vi "Post Webmessage.vi"(8 "error in (no error)":errorcluster, 9 "Send as JSON":bool, 10 "Message":string, 11 "WebView2 Control in":refnum<class "WebView2 Control.lvclass">) -> (0 "error out":errorcluster, 3 "WebView2 Control out":refnum<class "WebView2 Control.lvclass">)   [LabVIEW 2020, in "WebView2.lvlib" / "WebView2 Control.lvclass"]
uses:
  WebView2 Control.lvclass
  WebView2 Control.lvclass/WebView2 Control.ctl
  C:/Users/Simon/Documents/GitHub/LV-WebView2/Source/Libs/Microsoft.Web.WebView2.Core.dll
  Libs/Microsoft.Web.WebView2.Core.dll
  Read Core.vi
  Init WebView2 Core.vi
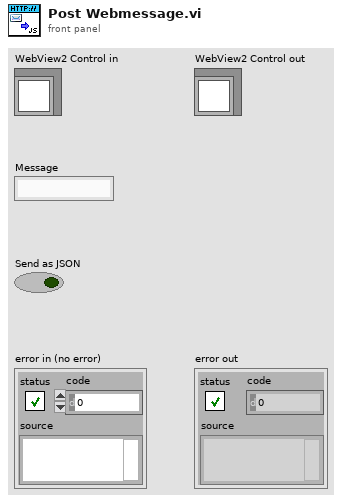
[diagram p1: front panel]
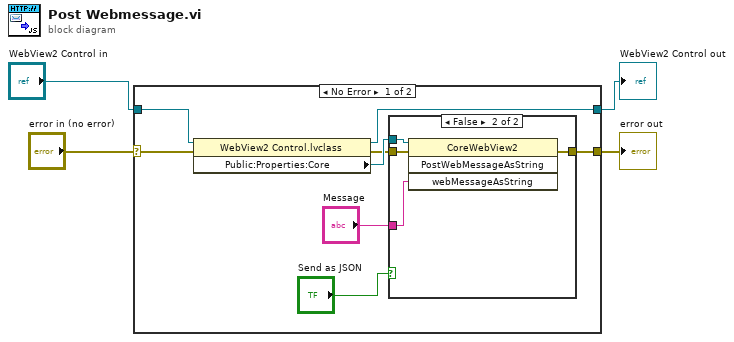
[diagram p0: block diagram]
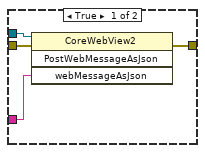
[diagram p2: hidden frame]
diagram:
  n1 = case shown="No Error" "error in (no error)" {
    selector: "error in (no error)" -> [w12 w22]
    tunnel: [w7 w22] -> w3
    tunnel: [w10 w21] -> w1
    tunnel: "WebView2 Control in" -> [w11 w21]
    frame No Error {
      n2 = property class="WebView2 Control.lvclass"(reference=w11, error in=w12) -> (reference out=w10:refnum<class "WebView2 Control.lvclass">, error out=w8:errorcluster, "Public:Properties:Core"=w9:refnum<k24>)
      n3 = case shown="False" "Send as JSON" {
        tunnel: w9 -> [w16 w20]
        tunnel: "Message" -> [w15 w19]
        tunnel: [w14 w18] -> w7
        tunnel: w8 -> [w13 w17]
        frame True {
          n4 = invoke class="CoreWebView2" method="PostWebMessageAsJson"(reference=w16, error in=w13, "webMessageAsJson"=w15) -> (error out=w14:errorcluster)  [unwired: 1 in, 3 out]
        }
        frame False {
          n5 = invoke class="CoreWebView2" method="PostWebMessageAsString"(reference=w20, error in=w17, "webMessageAsString"=w19) -> (error out=w18:errorcluster)  [unwired: 1 in, 3 out]
        }
      }
    }
    frame Error {
    }
  }
  "error out" <- w3
  "WebView2 Control out" <- w1
